vi "Read Parcel pickup address.vi"(8 "error in (no error)":errorcluster, 11 "Delivery in":refnum<class "Delivery.lvclass">) -> (0 "error out":errorcluster, 2 "Parcel pickup address":string, 3 "Delivery out":refnum<class "Delivery.lvclass">)   [LabVIEW 2019, in "Delivery.lvclass"]
uses:
  Delivery.lvclass
  Delivery.lvclass/Delivery.ctl
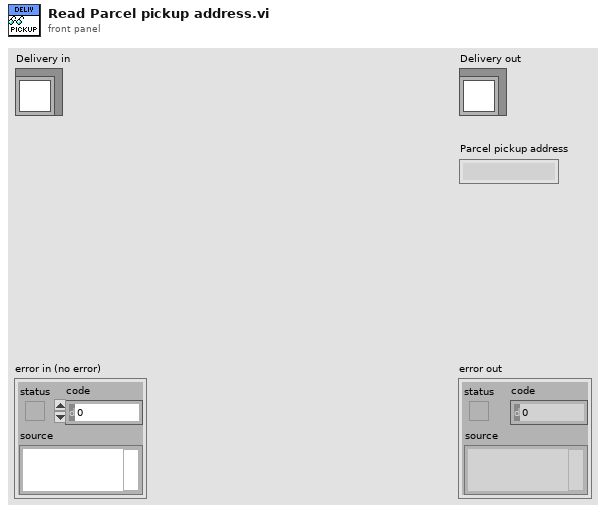
[diagram p1: front panel]
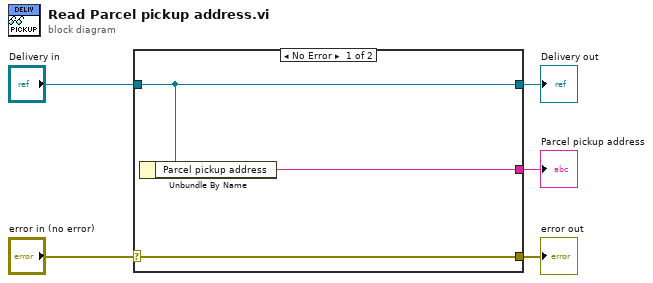
[diagram p0: block diagram]
diagram:
  n1 = case shown="No Error" "error in (no error)" {
    selector: "error in (no error)" -> [w8 w9]
    tunnel: [w8 w9] -> w4
    tunnel: [w7 w10] -> w2
    tunnel: "Delivery in" -> [w7 w10]
    tunnel: [w6 _] -> w1
    frame No Error {
      n2 = Unbundle By Name(w7) -> ("Parcel pickup address"=w6:string)
    }
    frame Error {
    }
  }
  "error out" <- w4
  "Delivery out" <- w2
  "Parcel pickup address" <- w1
